vi "Format Precision.vi"(8 "error in":errorcluster, 9 "Exponent":u16, 10 "Mantissa":u16, 11 "Instrument Handle In":i32) -> (0 "error out":errorcluster, 3 "Instrument Handle Out":i32)   [LabVIEW 8.6, in "ZTScopeM.lvlib"]
doc: "Configure the data precision for all floating point values from the instrument. The precision is specified in the following format:\n\nprecision = mantissa^exponent"
uses:
  ZTScopeM.lvlib
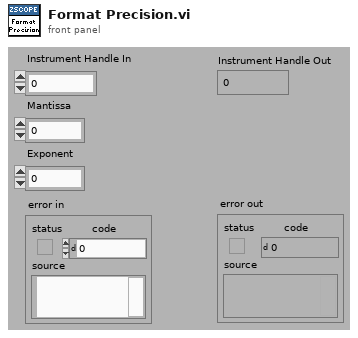
[diagram p1: front panel]
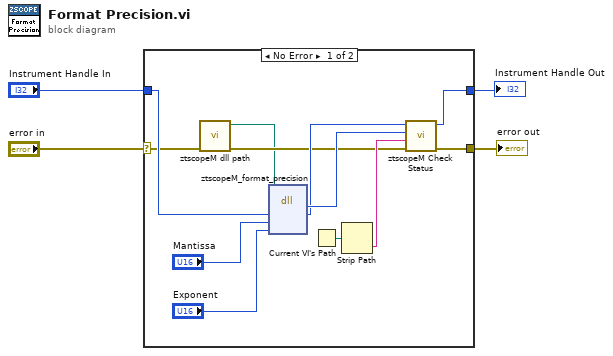
[diagram p0: block diagram]
diagram:
  n1 = case shown="No Error" "error in" {
    selector: "error in" -> [w6 w18]
    tunnel: [w9 w18] -> w1
    tunnel: "Instrument Handle In" -> [w16 w17]
    tunnel: [w8 w17] -> w3
    frame #0 {
      n2 = call "ztscopeM dll path.vi"("error in (no error)"=w6) -> ("error out"=w7:errorcluster, "<instrument>.dll path"=w5:path)  [unwired: 9 in]
      n3 = dll-call lib="C:/Program Files (x86)/National Instruments/LabVIEW 2013/instr.lib/ztscopem/ztscopeM.dll" fn="ztscopeM_format_precision"(path in=w5, "instrumentHandle"=w16, "mantissa"="Mantissa", "exponent"="Exponent") -> (w11:i32, "instrumentHandle"=w10:i32)  [unwired: 4 in, 2 out]
      n4 = Current VI's Path() -> (path=w13:path)
      n5 = Strip Path(path=w13) -> (name=w12:string)  [unwired: 1 out]
      n6 = call "ztscopeM Check Status.vi"("error in"=w7, "name of VI"=w12, "status (return code)"=w11, "instrument handle in"=w10) -> ("error out"=w9:errorcluster, "instrument handle out"=w8:i32)  [unwired: 2 in]
    }
    frame #1 {
    }
  }
  "Instrument Handle Out" <- w3
  "error out" <- w1
